vi "Assemble All Data file.vi"() -> (3 "All_Data Array":string[][](array[string]))   [LabVIEW 2013]
panel:
  in  "All_Data Bundle":T1={"Environment Details"=[["TI Automotive"], ["Caro Test Center"], ["628 Columbia St."], ["Caro, MI 48723"], [""], [""], [""]], "Instrument Identification"=[], "Standards Used"=[], "Calibration Details"=[], "Machine Specifications:"=[], "Channel Descriptions:"=[], "Tracking"=[], "CalChannelsAsFound"=[], "CalChannelsCalibrate"=[], "CalChannelsVerify"=[]}
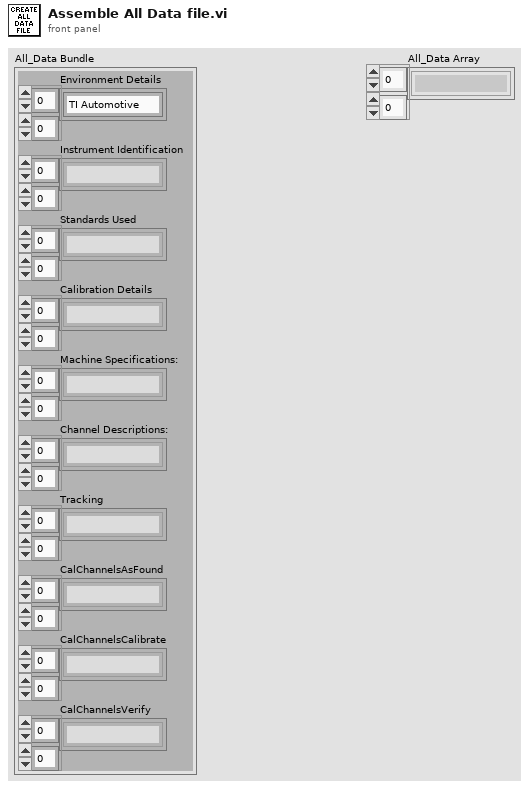
[diagram p1: front panel]
types:
  T1 = cluster{"Environment Details":string[][], "Instrument Identification":string[][], "Standards Used":string[][], "Calibration Details":string[][], "Machine Specifications:":string[][], "Channel Descriptions:":string[][], "Tracking":string[][], "CalChannelsAsFound":string[][], "CalChannelsCalibrate":string[][], "CalChannelsVerify":string[][]}
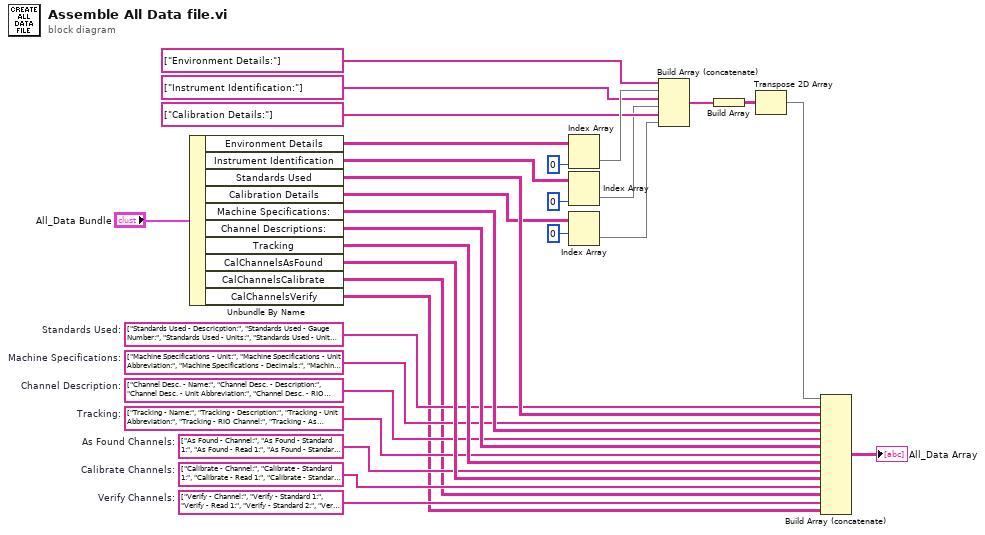
[diagram p0: block diagram]
diagram:
  w3 = string[] ["Verify - Channel:", "Verify - Standard 1:", "Verify - Read 1:", "Verify - Standard 2:", "Verify - Read 2:", "Verify - Standard 3:", "Verify - Read 3:", "Verify - Standard 4:", "Verify - Read 4:", "Verify - Standard 5:", "Verify - Read 5:"]  # Verify Channels:
  w4 = string[] ["Calibrate - Channel:", "Calibrate - Standard 1:", "Calibrate - Read 1:", "Calibrate - Standard 2:", "Calibrate - Read 2:", "Calibrate - Standard 3:", "Calibrate - Read 3:", "Calibrate - Standard 4:", "Calibrate - Read 4:", "Calibrate - Standard 5:", "Calibrate - Read 5:"]  # Calibrate Channels:
  w5 = string[] ["As Found - Channel:", "As Found - Standard 1:", "As Found - Read 1:", "As Found - Standard 2:", "As Found - Read 2:", "As Found - Standard 3:", "As Found - Read 3:", "As Found - Standard 4:", "As Found - Read 4:", "As Found - Standard 5:", "As Found - Read 5:"]  # As Found Channels:
  w29 = string[] ["Tracking - Name:", "Tracking - Description:", "Tracking - Unit Abbreviation:", "Tracking - RIO Channel:", "Tracking - As Found:", "Tracking - Calibrated:", "Tracking - Verified:"]  # Tracking:
  w27 = string[] ["Channel Desc. - Name:", "Channel Desc. - Description:", "Channel Desc. - Unit Abbreviation:", "Channel Desc. - RIO Channel:"]  # Channel Description:
  w25 = string[] ["Machine Specifications - Unit:", "Machine Specifications - Unit Abbreviation:", "Machine Specifications - Decimals:", "Machine Specifications - Min:", "Machine Specifications - Max:", "Machine Specifications - % Error(T)/Difference(F):", "Machine Specifications - Full Scale(T)/Teading(F)", "Machine Specifications - Tolerance Value:"]  # Machine Specifications:
  w23 = string[] ["Standards Used - Descricption:", "Standards Used - Gauge Number:", "Standards Used - Units:", "Standards Used - Unit Abbreviation:", "Standards Used - Calibration Due:"]  # Standards Used:
  n1 = Unbundle By Name("All_Data Bundle") -> ("Environment Details"=w22:string[][], "Instrument Identification"=w21:string[][], "Standards Used"=w24:string[][], "Calibration Details"=w20:string[][], "Machine Specifications:"=w26:string[][], "Channel Descriptions:"=w28:string[][], "Tracking"=w30:string[][], "CalChannelsAsFound"=w31:string[][], "CalChannelsCalibrate"=w2:string[][], "CalChannelsVerify"=w1:string[][])
  n2 = Index Array(array=w22, index (col)=0 ("disabled index (col)")) -> (element=w15:string[])  [unwired: 1 in]
  n3 = Index Array(array=w21, index (col)=0 ("disabled index (col)")) -> (element=w12:string[])  [unwired: 1 in]
  n4 = Index Array(array=w20, index (row)=0) -> (element=w11:string[])  [unwired: 1 in]
  n5 = Build Array (concatenate)(string[] ["Environment Details:"], w15, string[] ["Instrument Identification:"], w12, string[] ["Calibration Details:"], w11) -> (w10:string[])
  n6 = Build Array(w10) -> (w9:string[][])
  n7 = Transpose 2D Array(2D array=w9) -> (transposed array=w8:string[][])
  n8 = Build Array (concatenate)(w8, w23, w24, w25, w26, w27, w28, w29, w30, w5, w31, w4, w2, w3, w1) -> (→"All_Data Array":string[][])
